vi "Read terminalRef.vi"(8 "error in (no error)":errorcluster, 11 "Terminal In":refnum<class "Terminal.lvclass">) -> (0 "error out":errorcluster, 2 "terminalRef":refnum<vi>, 3 "Terminal Out":refnum<class "Terminal.lvclass">)   [LabVIEW 2023, in "TLC_Scripto.lvlib" / "Terminal.lvclass"]
uses:
  Terminal.lvclass
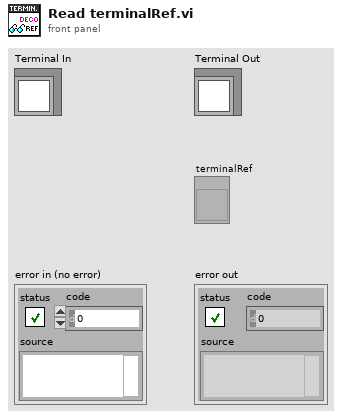
[diagram p1: front panel]
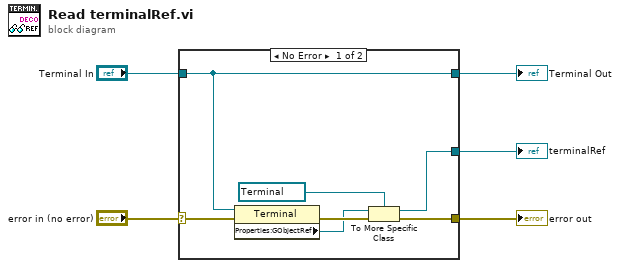
[diagram p0: block diagram]
diagram:
  n1 = case shown="No Error" "error in (no error)" {
    selector: "error in (no error)" -> [w8 w14]
    tunnel: [w7 w14] -> w4
    tunnel: [w9 w13] -> w2
    tunnel: "Terminal In" -> [w9 w13]
    tunnel: [w6 _] -> w1
    frame No Error {
      n2 = property class="Terminal"(reference=w9, error in=w8) -> (error out=w12:errorcluster, "Properties:GObjectRef"=w11:refnum<vi>)  [unwired: 1 out]
      n3 = To More Specific Class(target class=refnum<vi> refnum ("type"), reference=w11, error in=w12) -> (specific class reference=w6:refnum<vi>, error out=w7:errorcluster)
    }
    frame Error {
    }
  }
  "error out" <- w4
  "Terminal Out" <- w2
  "terminalRef" <- w1
